vi "ResetModuloCounters.vi"(8 "error in (no error)":errorcluster, 10 "Enum":enum16{"Slaves only", "Slaves & Master"}(ring), 11 "BME_DG_System in":refnum<class "BME_DG_System.lvclass">) -> (0 "error out":errorcluster, 3 "BME_DG_System out":refnum<class "BME_DG_System.lvclass">)   [LabVIEW 2009, in "POLARIS BME DG.lvlib" / "BME_DG_System.lvclass"]
uses:
  BME_DG_System.lvclass
  BME_DG_System.lvclass/BME_DG_System.ctl
  BME_DG_Base/BME_DG_Base.lvclass
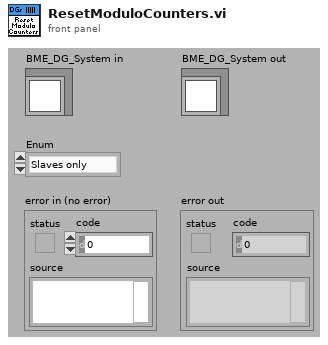
[diagram p1: front panel]
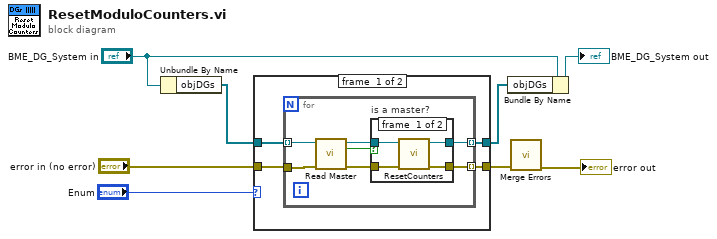
[diagram p0: block diagram]
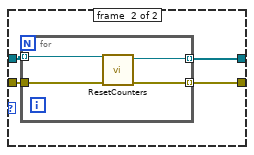
[diagram p3: hidden frame]
diagram:
  n1 = Unbundle By Name("BME_DG_System in") -> ("objDGs"=w3:refnum<class "BME_DG_Base.lvclass">[])
  n2 = case shown="\"Slaves & Master\"" "Enum" {
    tunnel: w3 -> [w12 w29]
    tunnel: "error in (no error)" -> [w11 w28]
    tunnel: [w10 w27] -> w2
    tunnel: [w9 w26] -> w1
    frame #0 {
      n3 = for {
        tunnel: w12 -> [w19] mode=indexing
        tunnel: w11 -> [w16]
        tunnel: [w14] -> w10 mode=indexing
        tunnel: [w13] -> w9 mode=indexing
        n4 = call-dynamic "Read Master.vi"("error in (no error)"=w16, "BME_DG_Base in"=w19) -> ("error out"=w17:errorcluster, "Master?"=w15:bool, "BME_DG_Base out"=w18:refnum<class "BME_DG_Base.lvclass">)  [unwired: 6 in, 1 out]
        n5 = case "is a master?" shown="False" w15 {
          tunnel: w18 -> [w23 w25]
          tunnel: w17 -> [w22 w24]
          tunnel: [w21 w25] -> w14
          tunnel: [w20 w24] -> w13
          frame #0 {
            n6 = call-dynamic "ResetCounters.vi"("error in (no error)"=w22, "BME_DG_Base in"=w23) -> ("error out"=w20:errorcluster, "BME_DG_Base out"=w21:refnum<class "BME_DG_Base.lvclass">)  [unwired: 8 in]
          }
          frame #1 {
          }
        }
      }
    }
    frame #1 {
      n7 = for {
        tunnel: w29 -> [w33] mode=indexing
        tunnel: w28 -> [w32]
        tunnel: [w31] -> w27 mode=indexing
        tunnel: [w30] -> w26 mode=indexing
        n8 = call-dynamic "ResetCounters.vi"("error in (no error)"=w32, "BME_DG_Base in"=w33) -> ("error out"=w30:errorcluster, "BME_DG_Base out"=w31:refnum<class "BME_DG_Base.lvclass">)  [unwired: 8 in]
      }
    }
  }
  n9 = Bundle By Name(cluster="BME_DG_System in", "objDGs"=w2) -> (→"BME_DG_System out":refnum<class "BME_DG_System.lvclass">)
  n10 = call <vilib>:"Merge Errors.vi"("error array in"=w1) -> ("error out"=→"error out":errorcluster)  [unwired: 6 in]
